vi "Save Calibration.vi"(8 "error in (no error)":errorcluster, 11 "PathControl in":refnum<class "PathControl.lvclass">) -> (0 "error out":errorcluster, 3 "PathControl out":refnum<class "PathControl.lvclass">)   [LabVIEW 2020, in "PathControl.lvclass"]
uses:
  PathControl.lvclass
  PathControl.lvclass/PathControl.ctl
  <vilib>/Utility/xml.llb/Write to XML File(string).vi
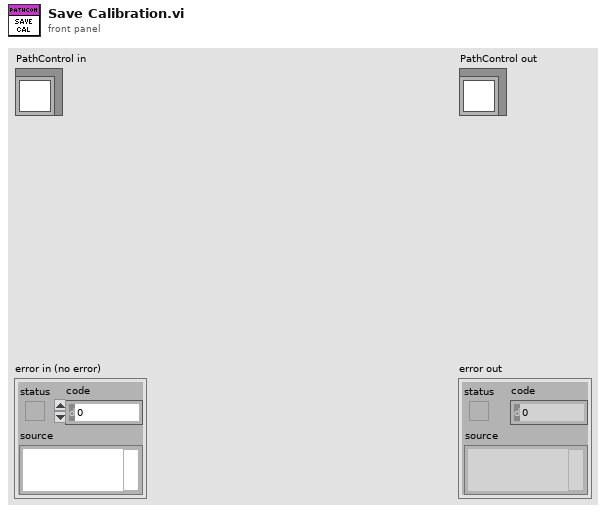
[diagram p1: front panel]
types:
  T1 = cluster{"Name":string, "Path Frequency":dbl[], "Path Loss":dbl[]}[]
  T2 = cluster{"Name":string, "Path Frequency":dbl[], "Path Loss":dbl[]}
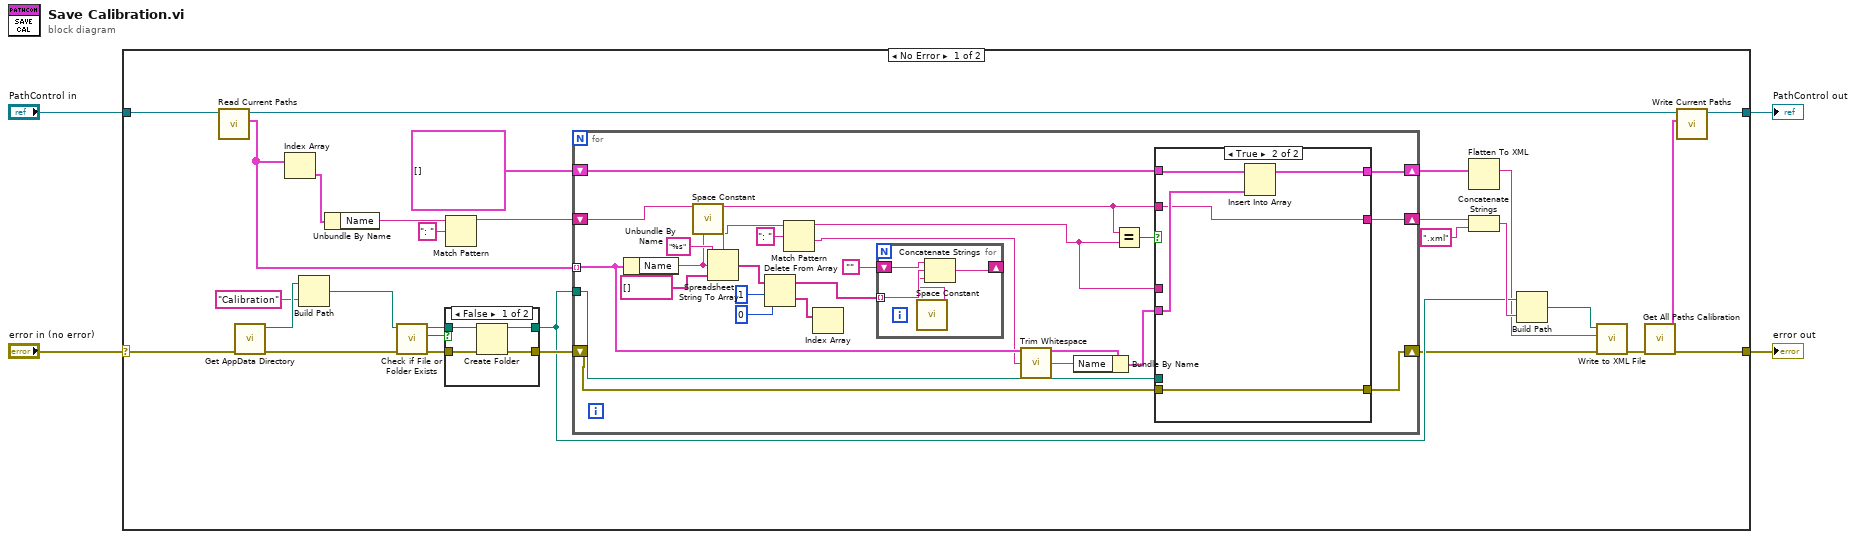
[diagram p0: block diagram]
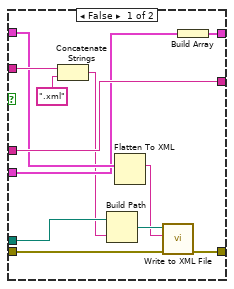
[diagram p3: hidden frame]
diagram:
  n1 = case shown="No Error" "error in (no error)" {
    selector: "error in (no error)" -> [w32 w86]
    tunnel: [w22 w86] -> w3
    tunnel: [w20 w85] -> w1
    tunnel: "PathControl in" -> [w33 w85]
    frame No Error {
      n2 = call "Read Current Paths.vi"("PathControl in"=w33) -> ("Current Paths"=w27:T1, "PathControl out"=w21:refnum<class "PathControl.lvclass">)  [unwired: 9 in]
      n3 = call "Get AppData Directory.vi"("Error In"=w32) -> ("Error Out"=w18:errorcluster, "Folder path"=w31:path)  [unwired: 8 in, 1 out]
      n4 = Index Array(array=w27) -> (element=w29:T2)  [unwired: 1 in]
      n5 = Build Path(base path=w31, name or relative path="Calibration") -> (appended path=w13:path)
      n6 = Unbundle By Name(w29) -> ("Name"=w6:string)
      n7 = call <vilib>:"Check if File or Folder Exists.vi"("error in (no error)"=w18, "path"=w13) -> ("error out"=w16:errorcluster, "file or folder exists?"=w17:bool, "dup path"=w15:path)  [unwired: 7 in]
      n8 = case shown="False" w17 {
        tunnel: w16 -> [w37 w39]
        tunnel: w15 -> [w36 w38]
        tunnel: [w35 w39] -> w14
        tunnel: [w34 w38] -> w12
        frame False {
          n9 = Create Folder(path (use dialog)=w36, error in=w37) -> (created path=w34:path, error out=w35:errorcluster)  [unwired: 1 in, 1 out]
        }
        frame True {
        }
      }
      n10 = Match Pattern(string=w6, regular expression=": ") -> (before substring=w5:string)  [unwired: 1 in, 3 out]
      n11 = for {
        tunnel: w12 -> [w49]
        tunnel: w27 -> [w55] mode=indexing
        shift-right: [w47] -> w26
        shift-left: w5 -> [w51]
        shift-right: [w50] -> w23
        shift-left: T1 [] ("Current Paths") -> [w52]
        shift-right: [w46] -> w8
        shift-left: w14 -> [w48]
        n12 = Unbundle By Name(w55) -> ("Name"=w43:string)
        n13 = call <vilib>:"Space Constant.vi"() -> ("String"=w62:string)
        n14 = Spreadsheet String To Array(delimiter (Tab)=w62, format string="%s", spreadsheet string=w43, array type (2D Dbl)=string[] []) -> (array=w60:string[])
        n15 = Delete From Array(array=w60, length=1, index=0) -> (deleted portion=w58:string[], array with subset deleted=w57:string[])
        n16 = Match Pattern(string=w43, regular expression=": ") -> (before substring=w41:string, after substring=w40:string)  [unwired: 1 in, 2 out]
        n17 = Index Array(array=w58) -> ()  [unwired: 1 in, 1 out]
        n18 = for {
          tunnel: w57 -> [w83] mode=indexing
          shift-right: [w81] -> _
          shift-left: "" -> [w84]
          n19 = call <vilib>:"Space Constant.vi"() -> ("String"=w82:string)
          n20 = Concatenate Strings(w84, w83, w82) -> (w81:string)
        }
        n21 = call <vilib>:"Trim Whitespace.vi"("string"=w40) -> ("trimmed string"=w44:string)  [unwired: 1 in]
        n22 = Bundle By Name(cluster=w55, "Name"=w44) -> (w53:T2)
        n23 = Equal?(x=w51, y=w41) -> (x = y?=w54:bool)
        n24 = case shown="True" w54 {
          tunnel: w53 -> [w71 w78]
          tunnel: w52 -> [w72 w80]
          tunnel: w51 -> [w74 w77]
          tunnel: w41 -> [w75 _]
          tunnel: [w70 w79] -> w50
          tunnel: w49 -> [w69 _]
          tunnel: w48 -> [w64 w76]
          tunnel: [w75 w77] -> w47
          tunnel: [w67 w76] -> w46
          frame False {
            n25 = Concatenate Strings(w74, ".xml" ("string")) -> (w68:string)
            n26 = Build Path(base path=w69, name or relative path=w68) -> (appended path=w66:path)
            n27 = Flatten To XML(6:w72) -> (2:w65:string)
            n28 = call-poly <vilib>:"Write to XML File.vi"("error in (no error)"=w64, "XML Input"=w65, "XML File Path"=w66) -> ("error out"=w67:errorcluster)  [unwired: 6 in, 2 out]
            n29 = Build Array(w71) -> (w70:T1)
          }
          frame True {
            n30 = Insert Into Array(array=w80, new element=w78) -> (w79:T1)  [unwired: 1 in]
          }
        }
      }
      n31 = Flatten To XML(6:w23) -> (2:w9:string)
      n32 = Concatenate Strings(w26, ".xml" ("string")) -> (w24:string)
      n33 = Build Path(base path=w12, name or relative path=w24) -> (appended path=w10:path)
      n34 = call-poly <vilib>:"Write to XML File.vi"("error in (no error)"=w8, "XML Input"=w9, "XML File Path"=w10) -> ("error out"=w11:errorcluster)  [unwired: 6 in, 2 out]
      n35 = call "Get All Paths Calibration.vi"("Error In"=w11) -> ("Error Out"=w22:errorcluster, "All Paths"=w19:T1)  [unwired: 9 in]
      n36 = call "Write Current Paths.vi"("Current Paths"=w19, "PathControl in"=w21) -> ("PathControl out"=w20:refnum<class "PathControl.lvclass">)  [unwired: 9 in]
    }
    frame Error {
    }
  }
  "error out" <- w3
  "PathControl out" <- w1
